vi "Create Brickwall Spectrum.vi"(8 "error in (no error)":errorcluster, 9 "Fs (Hz)":dbl=1.0 format="%#_13g", 10 "Npts":i32, 11 "Filter in":refnum<class "Filter.lvclass">) -> (0 "error out":errorcluster, 2 "Spectrum":dbl[](array[numeric]), 3 "Filter out":refnum<class "Filter.lvclass">)   [LabVIEW 2020, in "Filter.lvclass"]
uses:
  Filter.lvclass
  Filter.lvclass/Filter.ctl
  fb9fde12-ccc1-4a29-ad98-9597953da60b.vi
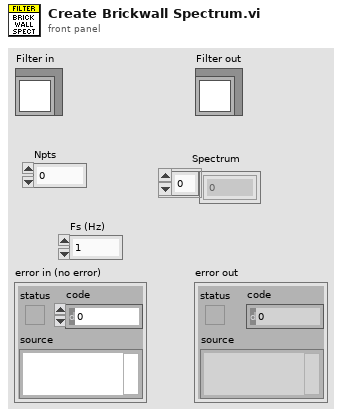
[diagram p1: front panel]
types:
  T1 = typedef "Filter.lvclass/Shape.ctl" = enum16{"OFF", "Lowpass", "Highpass", "Bandpass", "Bandstop"}
  T2 = typedef "Filter.lvclass/Units.ctl" = enum16{"Linear", "Octaves", "Min-Max"}
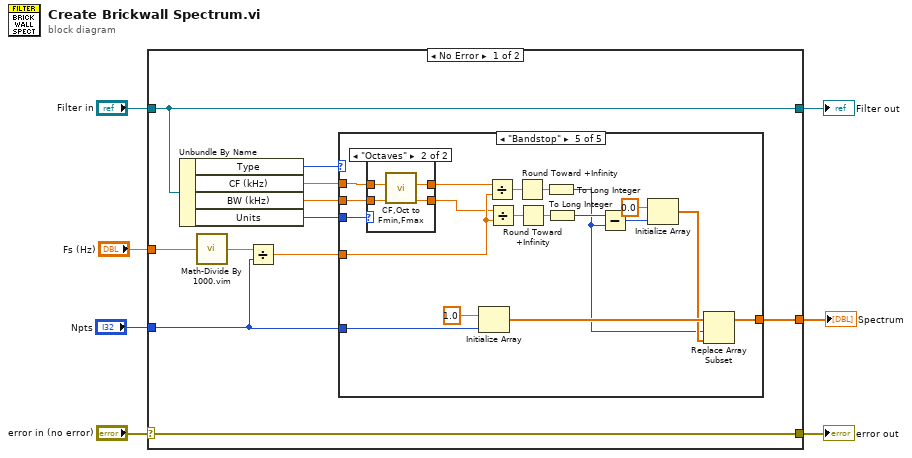
[diagram p0: block diagram]
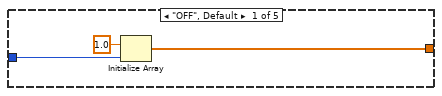
[diagram p2: hidden frame]
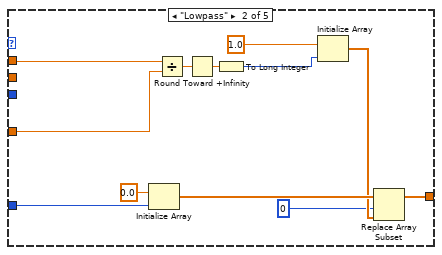
[diagram p3: hidden frame]
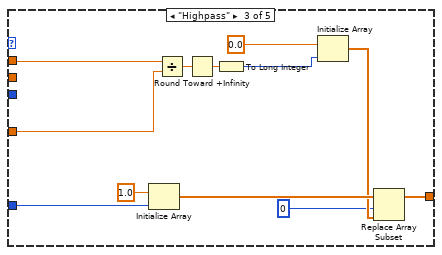
[diagram p4: hidden frame]
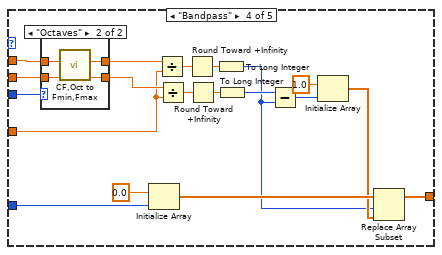
[diagram p5: hidden frame]
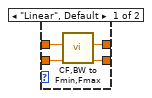
[diagram p6: hidden frame]
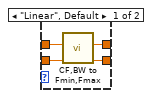
[diagram p7: hidden frame]
diagram:
  n1 = case shown="No Error" "error in (no error)" {
    selector: "error in (no error)" -> [w18 w101]
    tunnel: [w18 w101] -> w6
    tunnel: [w17 w100] -> w4
    tunnel: "Filter in" -> [w17 w100]
    tunnel: [w8 _] -> w3
    tunnel: "Fs (Hz)" -> [w13 _]
    tunnel: "Npts" -> [w9 _]
    frame No Error {
      n2 = Unbundle By Name(w17) -> ("Type"=w16:T1, "CF (kHz)"=w15:dbl, "BW (kHz)"=w14:dbl, "Units"=w10:T2)
      n3 = call "Math-Divide By 1000.vim"("X"=w13) -> ("1000X"=w11:dbl)
      n4 = Divide(x=w11, y=w9) -> (x/y=w12:dbl)
      n5 = case shown="\"Bandstop\"" w16 {
        tunnel: w9 -> [w21 w30 w42 w53 w84]
        tunnel: [w19 w28 w40 w51 w82] -> w8
        tunnel: w15 -> [_ w24 w36 w64 w77]
        tunnel: w14 -> [_ _ _ w63 w76]
        tunnel: w12 -> [_ w22 w34 w56 w87]
        tunnel: w10 -> [_ _ _ w46 w75]
        frame "OFF", Default {
          n6 = Initialize Array(1.0 ("element"), w21) -> (w19:dbl[])
        }
        frame "Lowpass" {
          n7 = Initialize Array(0.0 ("element"), w30) -> (w29:dbl[])
          n8 = Divide(x=w24, y=w22) -> (x/y=w32:dbl)
          n9 = Round Toward +Infinity(x=w32) -> (ceil(x): smallest int >= x=w33:dbl)
          n10 = To Long Integer(number=w33) -> (32bit integer=w25:i32)
          n11 = Initialize Array(1.0 ("element"), w25) -> (w26:dbl[])
          n12 = Replace Array Subset(array=w29, new element=w26, index=0) -> (w28:dbl[])
        }
        frame "Highpass" {
          n13 = Initialize Array(1.0 ("element"), w42) -> (w41:dbl[])
          n14 = Divide(x=w36, y=w34) -> (x/y=w44:dbl)
          n15 = Round Toward +Infinity(x=w44) -> (ceil(x): smallest int >= x=w45:dbl)
          n16 = To Long Integer(number=w45) -> (32bit integer=w37:i32)
          n17 = Initialize Array(0.0 ("element"), w37) -> (w38:dbl[])
          n18 = Replace Array Subset(array=w41, new element=w38, index=0) -> (w40:dbl[])
        }
        frame "Bandpass" {
          n19 = case shown="\"Octaves\"" w46 {
            tunnel: w64 -> [w68 w72]
            tunnel: w63 -> [w67 w71]
            tunnel: [w66 w70] -> w60
            tunnel: [w65 w69] -> w57
            frame "Linear", Default {
              n20 = call "CF,BW to Fmin,Fmax.vi"("BW"=w67, "CF"=w68) -> ("Fmax"=w65:dbl, "Fmin"=w66:dbl)  [unwired: 8 in]
            }
            frame "Octaves" {
              n21 = call "CF,Oct to Fmin,Fmax.vi"("BW"=w71, "CF"=w72) -> ("Fmax"=w69:dbl, "Fmin"=w70:dbl)  [unwired: 8 in]
            }
          }
          n22 = Initialize Array(0.0 ("element"), w53) -> (w52:dbl[])
          n23 = Divide(x=w60, y=w56) -> (x/y=w61:dbl)
          n24 = Divide(x=w57, y=w56) -> (x/y=w58:dbl)
          n25 = Round Toward +Infinity(x=w61) -> (ceil(x): smallest int >= x=w62:dbl)
          n26 = Round Toward +Infinity(x=w58) -> (ceil(x): smallest int >= x=w59:dbl)
          n27 = To Long Integer(number=w62) -> (32bit integer=w47:i32)
          n28 = To Long Integer(number=w59) -> (32bit integer=w55:i32)
          n29 = Subtract(x=w55, y=w47) -> (x-y=w50:i32)
          n30 = Initialize Array(1.0 ("element"), w50) -> (w48:dbl[])
          n31 = Replace Array Subset(array=w52, new element=w48, index=w47) -> (w51:dbl[])
        }
        frame "Bandstop" {
          n32 = case shown="\"Octaves\"" w75 {
            tunnel: w77 -> [w95 w99]
            tunnel: w76 -> [w94 w98]
            tunnel: [w93 w97] -> w74
            tunnel: [w92 w96] -> w73
            frame "Linear", Default {
              n33 = call "CF,BW to Fmin,Fmax.vi"("BW"=w94, "CF"=w95) -> ("Fmax"=w92:dbl, "Fmin"=w93:dbl)  [unwired: 8 in]
            }
            frame "Octaves" {
              n34 = call "CF,Oct to Fmin,Fmax.vi"("BW"=w98, "CF"=w99) -> ("Fmax"=w96:dbl, "Fmin"=w97:dbl)  [unwired: 8 in]
            }
          }
          n35 = Initialize Array(1.0 ("element"), w84) -> (w83:dbl[])
          n36 = Divide(x=w74, y=w87) -> (x/y=w90:dbl)
          n37 = Divide(x=w73, y=w87) -> (x/y=w88:dbl)
          n38 = Round Toward +Infinity(x=w90) -> (ceil(x): smallest int >= x=w91:dbl)
          n39 = Round Toward +Infinity(x=w88) -> (ceil(x): smallest int >= x=w89:dbl)
          n40 = To Long Integer(number=w91) -> (32bit integer=w78:i32)
          n41 = To Long Integer(number=w89) -> (32bit integer=w86:i32)
          n42 = Subtract(x=w86, y=w78) -> (x-y=w81:i32)
          n43 = Initialize Array(0.0 ("element"), w81) -> (w79:dbl[])
          n44 = Replace Array Subset(array=w83, new element=w79, index=w78) -> (w82:dbl[])
        }
      }
    }
    frame Error {
    }
  }
  "error out" <- w6
  "Filter out" <- w4
  "Spectrum" <- w3
